vi "From.vi"(1 "Value":path) -> (0 "Path":refnum<class "Path.lvclass">)   [LabVIEW 2018, in "Toolkit.lvlib" / "Data.lvlib" / "Path.lvclass"]
doc: "Wraps a LabVIEW path in a Mustache data type object."
uses:
  Path.lvclass
  Path.lvclass/Path.ctl
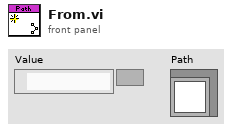
[diagram p1: front panel]
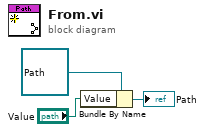
[diagram p0: block diagram]
diagram:
  n1 = Bundle By Name(cluster=refnum<class "Path.lvclass"> refnum ("Toolkit.lvlib:Data.lvlib:Path.lvclass"), "Value"="Value") -> (→"Path":refnum<class "Path.lvclass">)
